vi "writeCursors.vi"(9 "plotNumber":i32, 10 "dataCutCluster":refnum<vi>, 11 "WaveformGraph in":refnum<vi>) -> (2 "listOfProfiles":path[](array[path]), 3 "listOfProfiles":string[](array[string]))   [LabVIEW 2014]
uses:
  <vilib>/Utility/file.llb/Write To Spreadsheet File (string).vi
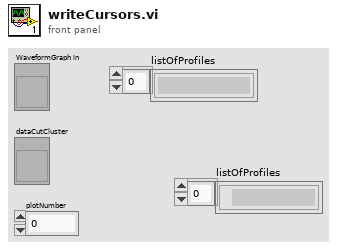
[diagram p1: front panel]
types:
  T1 = cluster{"data offset array":dbl[], "data cut array":waveform(dbl)[], "data lables":string[], "short data lables":string[]}
  T2 = typedef "LVCursorListTypeDef.ctl" = cluster{"Name":string, "Color":u32, "Style":u8, "Point Style":u8, "Name Visible":bool, "Allow Drag":bool, "Cursor Mode":u32, "Plot":i32, "Index":i32, "Position":cluster{"X":dbl, "Y":dbl}, "X Scale":u32, "Y Scale":u32, "Watch Plots":i32[], "Watch All Plots":bool, "Plot Area":i32, "Label Offset":cluster{"X":dbl, "Y":dbl}}[]
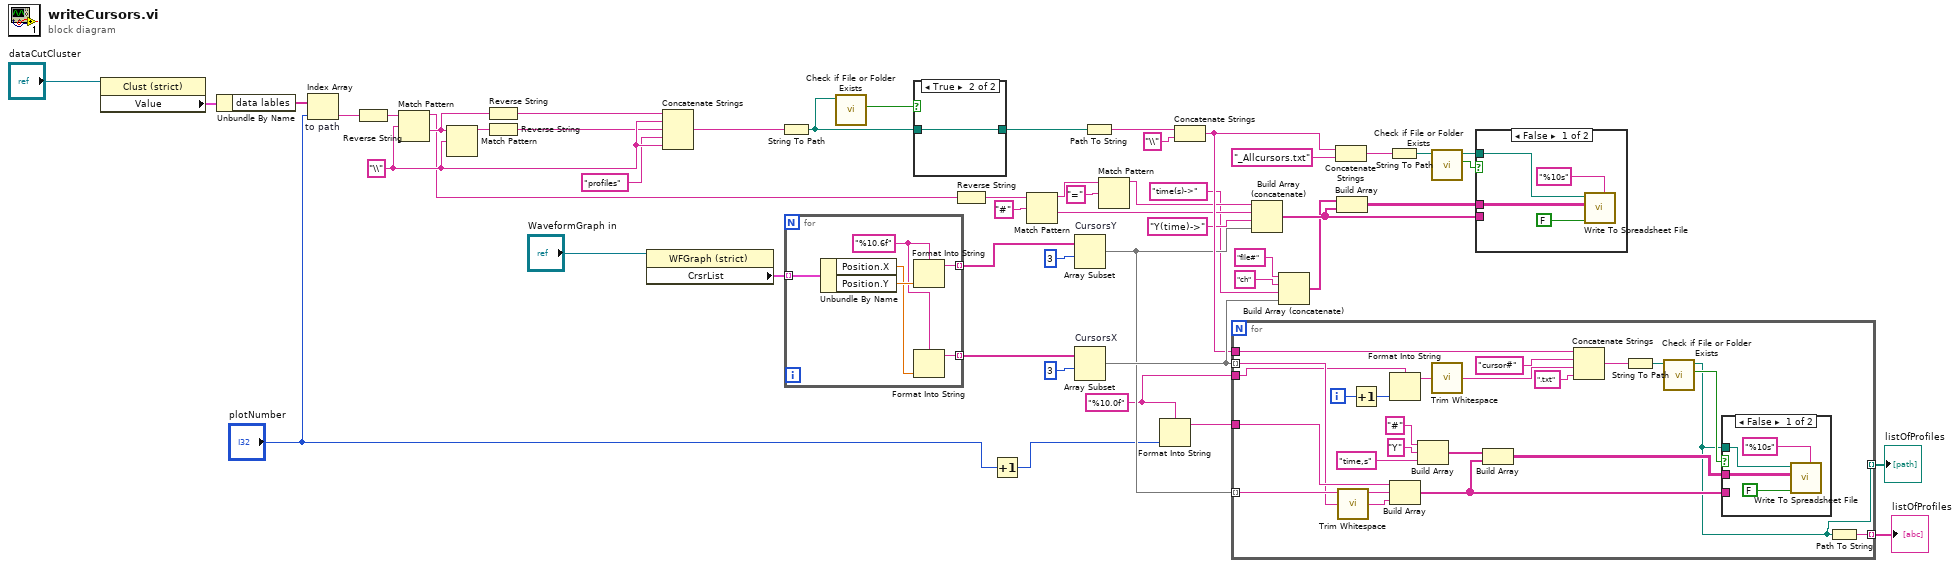
[diagram p0: block diagram]
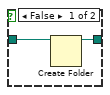
[diagram p2: hidden frame]
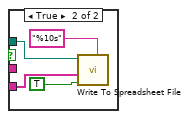
[diagram p3: hidden frame]
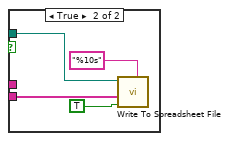
[diagram p4: hidden frame]
diagram:
  w4 = "%10.0f" ("format string")
  w40 = "\\" ("regular expression")
  n1 = property class="Clust (strict)"(reference="dataCutCluster") -> ("Value"=w27:T1)  [unwired: 1 in, 2 out]
  n2 = Unbundle By Name(w27) -> ("data lables"=w28:string[])
  n3 = Index Array "to path"(array=w28, index="plotNumber") -> (element=w9:string)
  n4 = Reverse String(1:w9) -> (0:w7:string)
  n5 = Match Pattern(string=w7, regular expression=w40) -> (before substring=w8:string, after substring=w10:string)  [unwired: 1 in, 2 out]
  n6 = Match Pattern(string=w10, regular expression=w40) -> (before substring=w11:string)  [unwired: 1 in, 3 out]
  n7 = Reverse String(1:w10) -> (0:w12:string)
  n8 = Reverse String(1:w11) -> (0:w39:string)
  n9 = property class="WFGraph (strict)"(reference="WaveformGraph in") -> ("CrsrList"=w17:T2)  [unwired: 1 in, 2 out]
  n10 = Concatenate Strings(w12, w40, w39, "profiles" ("string"), w40) -> (w41:string)
  n11 = String To Path(string=w41) -> (path=w43:path)
  n12 = for {
    tunnel: w17 -> [w57] mode=indexing
    tunnel: [w55] -> w18 mode=indexing
    tunnel: [w53] -> w49 mode=indexing
    w54 = "%10.6f" ("format string")
    n13 = Unbundle By Name(w57) -> ("Position.X"=w52:dbl, "Position.Y"=w56:dbl)
    n14 = Format Into String(format string=w54, w56) -> (resulting string=w55:string)  [unwired: 2 in, 1 out]
    n15 = Format Into String(format string=w54, w52) -> (resulting string=w53:string)  [unwired: 2 in, 1 out]
  }
  n16 = call <vilib>:"Check if File or Folder Exists.vi"("path"=w43) -> ("file or folder exists?"=w42:bool)  [unwired: 8 in, 2 out]
  n17 = case shown="True" w42 {
    tunnel: w43 -> [w59 w60]
    tunnel: [w58 w60] -> w44
    frame False {
      n18 = Create Folder(path (use dialog)=w59) -> (created path=w58:path)  [unwired: 2 in, 2 out]
    }
    frame True {
    }
  }
  n19 = Reverse String(1:w8) -> (0:w14:string)
  n20 = Increment(x="plotNumber") -> (x+1=w2:i32)
  n21 = Match Pattern(string=w14, regular expression="#") -> (before substring=w15:string, after substring=w34:string)  [unwired: 1 in, 2 out]
  n22 = Array Subset "CursorsY"(array=w18, index=3) -> (w36:string[])  [unwired: 1 in]
  n23 = Array Subset "CursorsX"(array=w49, index=3) -> (w51:string[])  [unwired: 1 in]
  n24 = Path To String(path=w44) -> (string=w45:string)
  n25 = Match Pattern(string=w15, regular expression="=") -> (before substring=w33:string)  [unwired: 1 in, 3 out]
  n26 = Format Into String(format string=w4, w2) -> (resulting string=w48:string)  [unwired: 2 in, 1 out]
  n27 = Concatenate Strings(w45, "\\" ("string")) -> (w47:string)
  n28 = for {
    tunnel: w47 -> [w83]
    tunnel: w36 -> [w78] mode=indexing
    tunnel: w48 -> [w77]
    tunnel: w51 -> [w75] mode=indexing
    tunnel: [w76] -> w37 mode=indexing
    tunnel: w4 -> [w73]
    tunnel: [w61] -> w1 mode=indexing
    i -> [w63]
    n29 = call <vilib>:"Trim Whitespace.vi"("string"=w75) -> ("trimmed string"=w72:string)  [unwired: 1 in]
    n30 = Increment(x=w63) -> (x+1=w62:i32)
    n31 = Format Into String(format string=w73, w62) -> (resulting string=w71:string)  [unwired: 2 in, 1 out]
    n32 = Build Array(w77, w78, w72) -> (w65:string[])
    n33 = Build Array("#", "Y", "time,s") -> (w66:string[])
    n34 = call <vilib>:"Trim Whitespace.vi"("string"=w71) -> ("trimmed string"=w70:string)  [unwired: 1 in]
    n35 = Build Array(w66, w65) -> (w64:string[][])
    n36 = Concatenate Strings(w83, "cursor#" ("string"), w70, ".txt" ("string")) -> (w80:string)
    n37 = String To Path(string=w80) -> (path=w81:path)
    n38 = call <vilib>:"Check if File or Folder Exists.vi"("path"=w81) -> ("file or folder exists?"=w79:bool, "dup path"=w61:path)  [unwired: 8 in, 1 out]
    n39 = case shown="False" w79 {
      tunnel: w61 -> [w87 w88]
      tunnel: w65 -> [_ w89]
      tunnel: w64 -> [w84 _]
      frame False {
        n40 = call-poly <vilib>:"Write To Spreadsheet File.vi"("format (%s)"="%10s" ("format string"), "append to file? (new file:F)"=FALSE ("transpose? (no:F)"), "2D data"=w84, "file path (dialog if empty)"=w87) -> ()  [unwired: 4 in, 1 out]
      }
      frame True {
        n41 = call-poly <vilib>:"Write To Spreadsheet File.vi"("format (%s)"="%10s" ("format string"), "append to file? (new file:F)"=TRUE ("transpose? (no:F)"), "1D data"=w89, "file path (dialog if empty)"=w88) -> ()  [unwired: 4 in, 1 out]
      }
    }
    n42 = Path To String(path=w61) -> (string=w76:string)
  }
  "listOfProfiles" <- w37
  "listOfProfiles" <- w1
  n43 = Build Array (concatenate)(w33, w34, "Y(time)->" ("element"), w36) -> (w21:string[])
  n44 = Build Array (concatenate)("file#", "ch" ("element"), "time(s)->" ("element"), w51) -> (w20:string[])
  n45 = Concatenate Strings(w47, "_Allcursors.txt") -> (w31:string)
  n46 = Build Array(w20, w21) -> (w22:string[][])
  n47 = String To Path(string=w31) -> (path=w19:path)
  n48 = call <vilib>:"Check if File or Folder Exists.vi"("path"=w19) -> ("file or folder exists?"=w5:bool, "dup path"=w6:path)  [unwired: 8 in, 1 out]
  n49 = case shown="False" w5 {
    tunnel: w6 -> [w95 w96]
    tunnel: w21 -> [_ w97]
    tunnel: w22 -> [w94 _]
    frame False {
      n50 = call-poly <vilib>:"Write To Spreadsheet File.vi"("format (%s)"="%10s", "append to file? (new file:F)"=FALSE ("transpose? (no:F)"), "2D data"=w94, "file path (dialog if empty)"=w95) -> ()  [unwired: 4 in, 1 out]
    }
    frame True {
      n51 = call-poly <vilib>:"Write To Spreadsheet File.vi"("format (%s)"="%10s" ("format string"), "append to file? (new file:F)"=TRUE ("transpose? (no:F)"), "1D data"=w97, "file path (dialog if empty)"=w96) -> ()  [unwired: 4 in, 1 out]
    }
  }
